vi "Set Protocol.vi"(8 "error in (no error)":errorcluster, 10 "Protocol":T1=1 items=["Sftp", "Scp", "Ftp", "Webdav", "S3"], 11 "SessionOptions in":refnum<class "SessionOptions.lvclass">) -> (0 "error out":errorcluster, 3 "SessionOptions out":refnum<class "SessionOptions.lvclass">)   [LabVIEW 2015, in "WinSCP.lvlib" / "SessionOptions.lvclass"]
uses:
  SessionOptions.lvclass
  Protocols--Ring.ctl
  SessionOptions.lvclass/SessionOptions.ctl
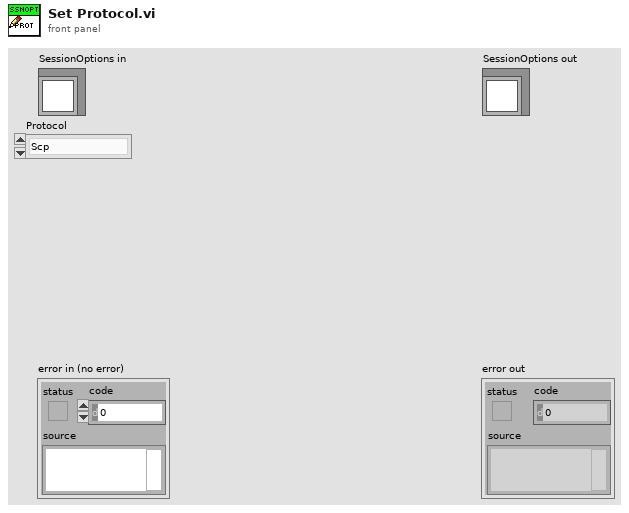
[diagram p1: front panel]
types:
  T1 = typedef "WinSCP.lvlib/SessionOptions.lvclass/Protocols--Ring.ctl" = i32
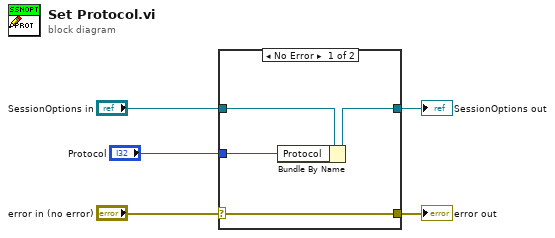
[diagram p0: block diagram]
diagram:
  n1 = case shown="No Error" "error in (no error)" {
    selector: "error in (no error)" -> [w8 w11]
    tunnel: [w8 w11] -> w4
    tunnel: [w7 w10] -> w2
    tunnel: "SessionOptions in" -> [w9 w10]
    tunnel: "Protocol" -> [w6 _]
    frame No Error {
      n2 = Bundle By Name(cluster=w9, "Protocol"=w6) -> (w7:refnum<class "SessionOptions.lvclass">)
    }
    frame Error {
    }
  }
  "error out" <- w4
  "SessionOptions out" <- w2
